vi "Check sweep timing.vi"(8 "error in (no error)":errorcluster, 10 "Tolerance (s)":dbl, 11 "DAQOrcaFlash in":refnum<class "DAQOrcaFlash.lvclass">) -> (0 "error out":errorcluster, 2 "out of time?":bool, 3 "DAQOrcaFlash out":refnum<class "DAQOrcaFlash.lvclass">)   [LabVIEW 2012, in "DAQOrcaFlash.lvclass"]
uses:
  DAQOrcaFlash.lvclass
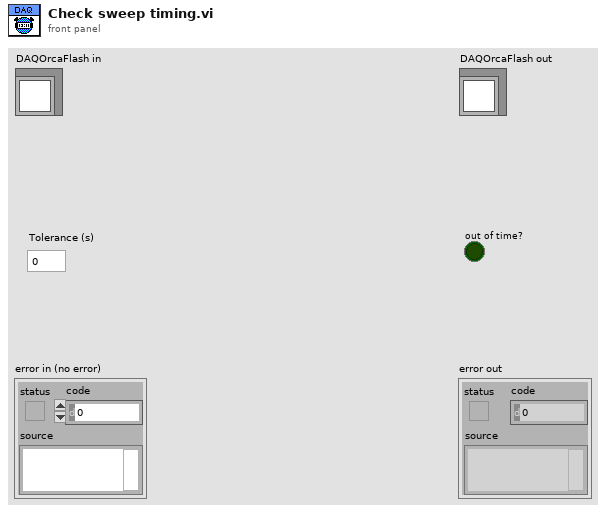
[diagram p1: front panel]
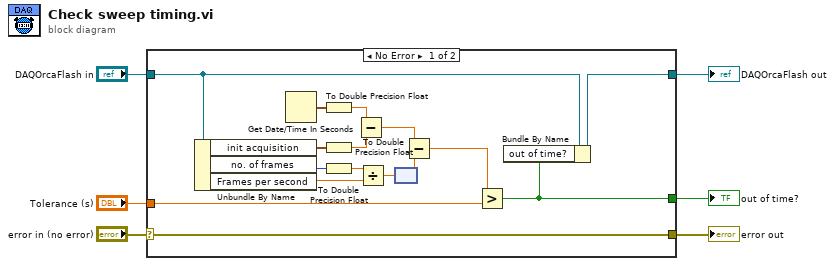
[diagram p0: block diagram]
diagram:
  n1 = case shown="No Error" "error in (no error)" {
    selector: "error in (no error)" -> [w22 w24]
    tunnel: [w22 w24] -> w5
    tunnel: [w8 w23] -> w3
    tunnel: "DAQOrcaFlash in" -> [w9 w23]
    tunnel: "Tolerance (s)" -> [w11 _]
    tunnel: [w7 _] -> w1
    frame No Error {
      n2 = Unbundle By Name(w9) -> ("init acquisition"=w18:timestamp, "no. of frames"=w21:i32, "Frames per second"=w20:dbl[unit])
      n3 = Get Date/Time In Seconds() -> (seconds since 1Jan1904=w17:timestamp)
      n4 = To Double Precision Float(number=w17) -> (double precision float=w16:dbl)
      n5 = To Double Precision Float(number=w18) -> (double precision float=w15:dbl)
      n6 = To Double Precision Float(number=w21) -> (double precision float=w19:dbl)
      n7 = Subtract(x=w16, y=w15) -> (x-y=w14:dbl)
      n8 = Divide(x=w19, y=w20) -> (x/y=w13:dbl[unit])
      n9 = node(w13) -> (w12:dbl)
      n10 = Subtract(x=w14, y=w12) -> (x-y=w10:dbl)
      n11 = Greater?(x=w10, y=w11) -> (0:w7:bool)
      n12 = Bundle By Name(cluster=w9, "out of time?"=w7) -> (w8:refnum<class "DAQOrcaFlash.lvclass">)
    }
    frame Error {
    }
  }
  "error out" <- w5
  "DAQOrcaFlash out" <- w3
  "out of time?" <- w1
